vi "Subtract.vi"(10 "y":dbl, 11 "x":dbl) -> (3 "x-y":dbl)   [LabVIEW 2023]
doc: "Use the LabVIEW Unit Test Framework Toolkit to check this VI for functional correctness. The test file for this VI, Subtract.lvtest, is configured to fail."
panel:
  # "Overview: Use the LabVIEW Unit Test Framework Toolkit to check this VI for functional correctness.\nRequirements: LabVIEW Full Development System, Unit Test Framework Toolkit\nInstructions:\n1.  Execute the Subtract.lvtest test file for this VI. In the Project Explorer window, expand the Unit Test Files folder, right-click Subtract.lvtest, and select Run from the shortcut menu.\n2.  View the test results in the Unit Test Frameworks Results window, which shows that this test fails."
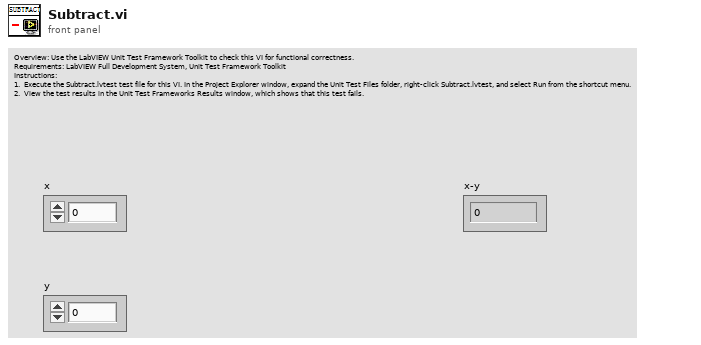
[diagram p1: front panel]
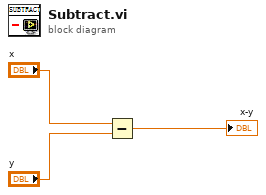
[diagram p0: block diagram]
diagram:
  n1 = Subtract(x="x", y="y") -> (x-y=→"x-y":dbl)
